vi "conv2matV2_old.vi"(0 "Ref Num":refnum<file>, 1 "Array name":string, 5 "pos mode (rel. to end: 1)":i16(ring)=1 items=["relative to beginning of file", "relative to end of file", "relative to current mark"], 7 "pos offset (bytes:0)":i32, 11 "error in (no error)":errorcluster, 12 "1D-array":dbl[](array[numeric]) min=0.0 max=127.0 format="%.2f") -> (4 "Dup Ref Num":refnum<file>, 8 "mark after write (bytes)":i32, 15 "error out":errorcluster)   [LabVIEW 2015]
doc: "CONV2MAT.VI exports an array to Matlab format (.MAT file) at the specified location. The default location is at the end of file. The user will have to open the output file before and close it afterwards. The VI does incoming and internal error checking and does not write if an incoming error occurs.\n\nConnect the following terminals:\n- Ref number\n- array name; this name will also apear when the resulting file is read\n into Matlab.\n- Data type; this specifies the output data type. This can come in\n handy if you want to reduce the output file size.\n- either 1D-array, 2D-array or String. If you want to write a string,\n do not connect Data Type (caracters will be converted to floating\n point numbers representing their ASCII-value).\n\nPos mode and Pos offset default to write any data at the end of the file.\n\nAlbert K. Wijnja\nUniversity of Technology Eindhoven\nE-mail: albert@wfw.wtb.tue.nl\n\nSeptember 1994"
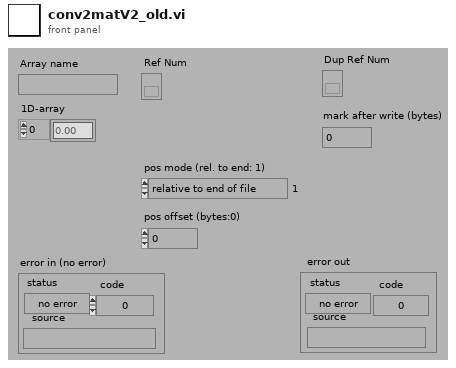
[diagram p1: front panel]
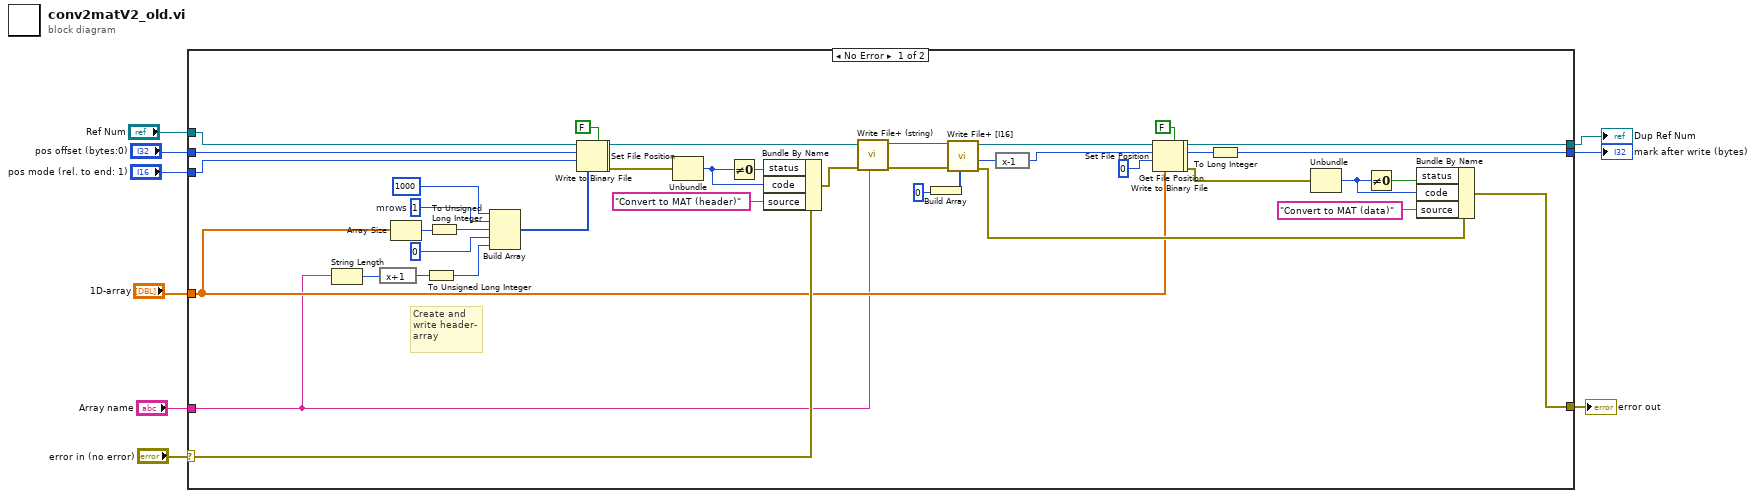
[diagram p0: block diagram]
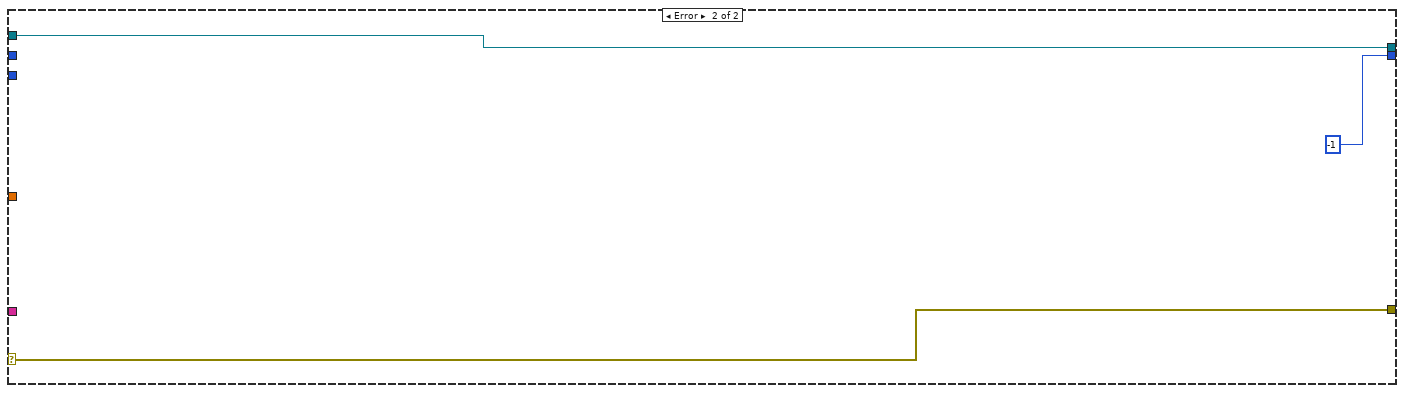
[diagram p2: hidden frame]
diagram:
  n1 = case shown="No Error" "error in (no error)" {
    selector: "error in (no error)" -> [w20 w56]
    tunnel: [w40 w56] -> w9
    tunnel: [w37 w58] -> w7
    tunnel: "Ref Num" -> [w47 w58]
    tunnel: [w36 -1] -> w6
    tunnel: "1D-array" -> [w17 _]
    tunnel: "Array name" -> [w16 _]
    tunnel: "pos offset (bytes:0)" -> [w13 _]
    tunnel: "pos mode (rel. to end: 1)" -> [w12 _]
    frame No Error {
      w34 = u32 1  # mrows
      # "Create and\nwrite header-\narray"
      n2 = String Length(string=w16) -> (length=w15:i32)
      n3 = expression code="x+1"(w15) -> (w14:i32)
      n4 = Array Size ("ncols")(array=w17) -> (size(s)=w21:i32)
      n5 = To Unsigned Long Integer(number=w14) -> (unsigned 32bit integer=w53:u32)
      n6 = To Unsigned Long Integer(number=w21) -> (unsigned 32bit integer=w33:u32)
      n7 = Build Array(u32 1000, w34, w33, u32 0, w53) -> (w46:u32[])
      n8 = Set File Position(offset (in bytes) (0)=w13, refnum=w47) -> (refnum out=w31:refnum<file>, error out=w30:errorcluster)  [unwired: 2 in]
      n9 = Write to Binary File(file (use dialog)=w31, data=w46, error in=w30, 5:FALSE ("prepend array or string size? (T)"), 9:w12) -> (refnum out=w52:refnum<file>, error out=w45:errorcluster)  [unwired: 1 in, 1 out]
      n10 = Unbundle(w45) -> ("code"=w32:i32)  [unwired: 2 out]
      n11 = Not Equal To 0?(x=w32) -> (x != 0?=w55:bool)
      n12 = Bundle By Name(cluster=w20, "status"=w55, "code"=w32, "source"="Convert to MAT (header)") -> (w44:errorcluster)
      n13 = call <vilib>:"Write File+ (string).vi"("string"=w16, "error in (no error)"=w44, "refnum"=w52) -> ("error out"=w49:errorcluster, "dup refnum"=w48:refnum<file>)  [unwired: 4 in, 1 out]
      n14 = Build Array(u8 0) -> (w51:u8[])
      n15 = call <vilib>:"Write File+ [I16].vi"("1D array"=w51, "error in (no error)"=w49, "refnum"=w48) -> ("error out"=w41:errorcluster, "mark after write (bytes)"=w11:i32, "dup refnum"=w38:refnum<file>)  [unwired: 6 in]
      n16 = expression code="x-1"(w11) -> (w10:i32)
      n17 = Set File Position(offset (in bytes) (0)=w10, refnum=w38, from (0:start)=i16 0) -> (refnum out=w27:refnum<file>, error out=w26:errorcluster)  [unwired: 1 in]
      n18 = Write to Binary File(file (use dialog)=w27, data=w17, error in=w26, 5:FALSE ("prepend array or string size? (T)")) -> (refnum out=w25:refnum<file>, error out=w24:errorcluster)  [unwired: 2 in, 1 out]
      n19 = Get File Position(4:w24, 7:w25) -> (0:w28:errorcluster, 2:w23:i64, 3:w37:refnum<file>)
      n20 = To Long Integer(number=w23) -> (32bit integer=w36:i32)
      n21 = Unbundle(w28) -> ("code"=w35:i32)  [unwired: 2 out]
      n22 = Not Equal To 0?(x=w35) -> (x != 0?=w42:bool)
      n23 = Bundle By Name(cluster=w41, "status"=w42, "code"=w35, "source"="Convert to MAT (data)") -> (w40:errorcluster)
    }
    frame Error {
    }
  }
  "Dup Ref Num" <- w7
  "error out" <- w9
  "mark after write (bytes)" <- w6
